vi "IPI_Cal_X_index_Pos_Step3.vi"(9 "mm":sgl, 10 "X pos":dbl[](array[numeric]), 11 "Axis Radio":T1) -> (3 "result X pos":dbl[](array[numeric]))   [LabVIEW 2015]
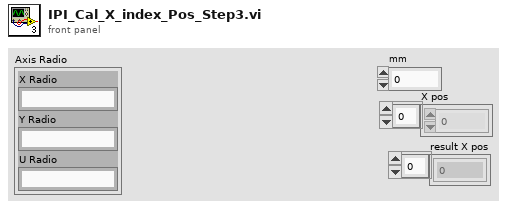
[diagram p1: front panel]
types:
  T1 = cluster{"X Radio":string, "Y Radio":string, "U Radio":string}
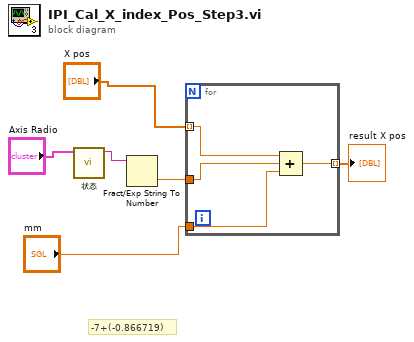
[diagram p0: block diagram]
diagram:
  # "-7+(-0.866719)"
  n1 = call "状态.vi"("Axis Radio"="Axis Radio") -> ("Axis X Postion"=w5:string)  [unwired: 6 in, 4 out]
  n2 = Fract/Exp String To Number(string=w5) -> (number=w4:dbl)  [unwired: 3 in, 1 out]
  n3 = for {
    tunnel: "X pos" -> [w10] mode=indexing
    tunnel: w4 -> [w9]
    tunnel: "mm" -> [w8]
    tunnel: [w7] -> w2 mode=indexing
    n4 = Compound Arithmetic op=ADD(w10, w9, w8) -> (w7:dbl)
  }
  "result X pos" <- w2
